vi "CurrentOutput_FBL.vi"(7 "y scaled":dbl, 9 "array":dbl[][](array[numeric]), 10 "Z Input":dbl, 11 "X Input":dbl) -> (0 "Origin":dbl, 1 "FW":dbl, 2 "FH":dbl, 3 "Current Out (pA)":dbl, 4 "Zread":dbl)   [LabVIEW 2017]
uses:
  <vilib>/ptbypt/NI_PtbyPt.lvlib
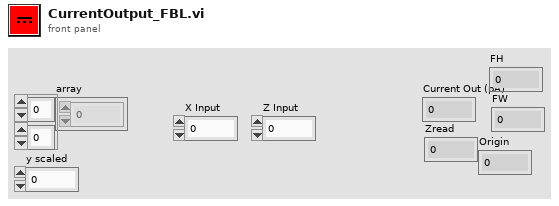
[diagram p1: front panel]
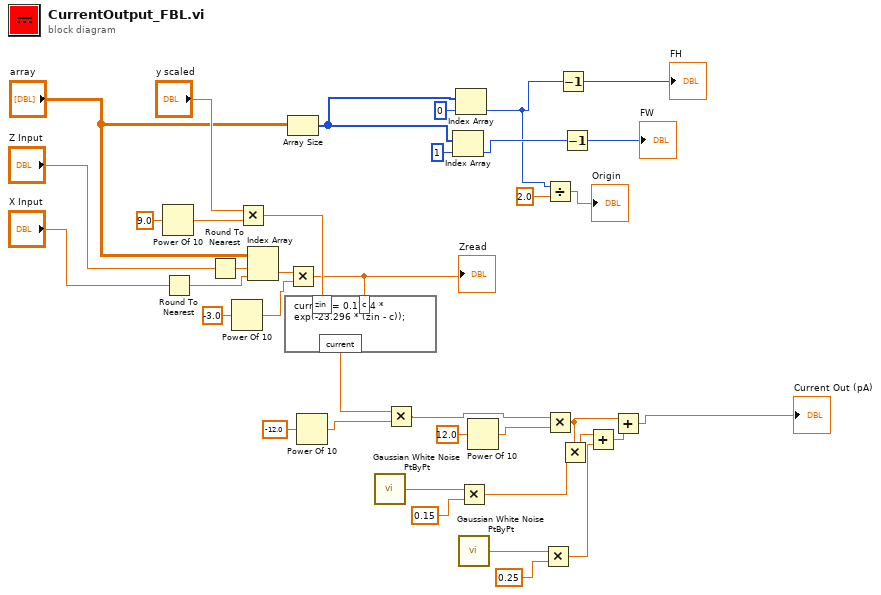
[diagram p0: block diagram]
diagram:
  n1 = Power Of 10(x=9.0) -> (10^x=w34:dbl)
  n2 = Round To Nearest(number="X Input") -> (nearest integer value=w28:dbl)
  n3 = Round To Nearest(number="Z Input") -> (nearest integer value=w36:dbl)
  n4 = Power Of 10(x=-3.0) -> (10^x=w30:dbl)
  n5 = Multiply(x="y scaled", y=w34) -> (x*y=w32:dbl)
  n6 = Index Array(array="array", index (row)=w36, index (col)=w28) -> (element=w25:dbl)
  n7 = Array Size(array="array") -> (size(s)=w20:i32[])
  n8 = Multiply(x=w25, y=w30) -> (x*y=w29:dbl)
  "Zread" <- w29
  n9 = formula code="current = 0.1714 * exp(-23.296 * (zin - c));"("zin"=w32, "c"=w29) -> ("current"=w35:dbl)
  n10 = Power Of 10(x=-12.0) -> (10^x=w38:dbl)
  n11 = call <vilib>:"Gaussian White Noise PtByPt.vi"() -> ("Gaussian white noise"=w11:dbl)  [unwired: 3 in]
  n12 = Multiply(x=w35, y=w38) -> (x*y=w2:dbl)
  n13 = Index Array(array=w20, index=1) -> (element=w19:i32)
  n14 = Index Array(array=w20, index=0) -> (element=w17:i32)
  n15 = Multiply(x=w11, y=0.15) -> (x*y=w9:dbl)
  n16 = call <vilib>:"Gaussian White Noise PtByPt.vi"() -> ("Gaussian white noise"=w7:dbl)  [unwired: 3 in]
  n17 = Power Of 10(x=12.0) -> (10^x=w13:dbl)
  n18 = Multiply(x=w7, y=0.25) -> (x*y=w3:dbl)
  n19 = Divide(x=w17, y=2.0) -> (x/y=→"Origin":dbl)
  n20 = Multiply(x=w2, y=w13) -> (x*y=w8:dbl)
  n21 = Decrement(x=w17) -> (x-1=→"FH":i32)
  n22 = Multiply(x=w8, y=w9) -> (x*y=w4:dbl)
  n23 = Decrement(x=w19) -> (x-1=→"FW":i32)
  n24 = Add(x=w4, y=w3) -> (x+y=w5:dbl)
  n25 = Add(x=w8, y=w5) -> (x+y=→"Current Out (pA)":dbl)
